vi "Get Status.vi"(8 "error in (no error)":errorcluster, 11 "IContainer in":refnum<class "IContainer.lvclass">) -> (0 "error out":errorcluster, 2 "Status":string, 3 "IContainer out":refnum<class "IContainer.lvclass">)   [LabVIEW 2013, in "IContainer.lvclass"]
doc: "Copyright 2018, Wiebe Walstra, wiebe@carya.nl."
uses:
  IContainer.lvclass
  IObject.lvclass
  IContainer.lvclass/IContainer.ctl
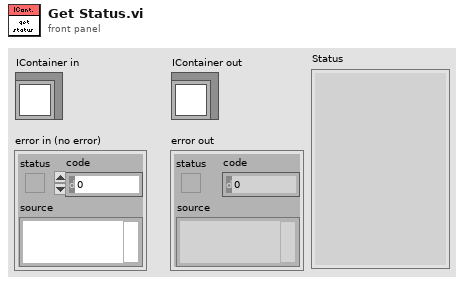
[diagram p1: front panel]
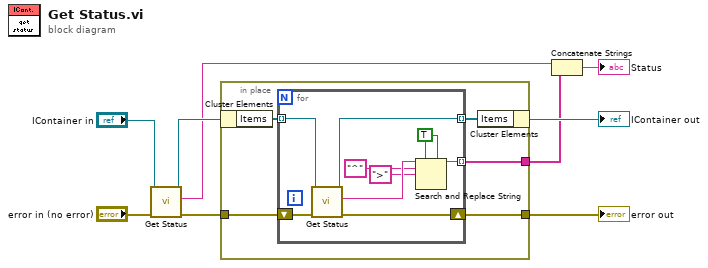
[diagram p0: block diagram]
diagram:
  n1 = call-parent "Get Status.vi"("error in (no error)"="error in (no error)", "IObject in"="IContainer in") -> ("error out"=w7:errorcluster, "Status"=w2:string, "IObject out"=w5:refnum<class "IContainer.lvclass">)  [unwired: 7 in]
  n2 = in-place {
    in-place-border: [w13] -> w6
    in-place-border: w7 -> [w12]
    in-place-border: [w10] -> w3
    n3 = in-place-cluster #1(w5) -> ("Items"=w11:refnum<class "IObject.lvclass">[])
    n4 = for {
      tunnel: [w22] -> w14 mode=indexing
      tunnel: w11 -> [w21] mode=indexing
      shift-right: [w23] -> w13
      shift-left: w12 -> [w20]
      tunnel: [w19] -> w10 mode=indexing
      w15 = TRUE ("replace all? (F)")
      n5 = call-dynamic "Get Status.vi"("error in (no error)"=w20, "IObject in"=w21) -> ("error out"=w23:errorcluster, "Status"=w18:string, "IObject out"=w22:refnum<class "IObject.lvclass">)  [unwired: 7 in]
      n6 = Search and Replace String(replace all?=w15, multiline?=w15, input string=w18, search string="^", replace string=">" ("replace string (\"\")")) -> (result string=w19:string)  [unwired: 3 in, 3 out]
    }
    n7 = in-place-cluster #1("Items"=w14) -> (→"IContainer out":refnum<class "IContainer.lvclass">)
  }
  "error out" <- w6
  n8 = Concatenate Strings(w2, w3) -> (→"Status":string)
